vi "AlliGator Save Phasor Ratio References.vi"(8 "Error In":errorcluster) -> (0 "Error Out":errorcluster, 1 "Message":string)   [LabVIEW 2021, in "AlliGator Phasor Ratio.lvlib"]
doc: "Saves phasor reference(s) - with Dialog."
uses:
  AlliGator Phasor Ratio.lvlib
  AlliGator Phasor Ratio Reference & Lifetime v2.ctl
  Phasor/Phasor (g, s).ctl
  Phasor/Phasor.lvlib
  Files/Files.lvlib
panel:
  in  "Cancel":bool
  in  "Save":bool
  in  "Save Reference 2":bool
  in  "Save Reference 1":bool
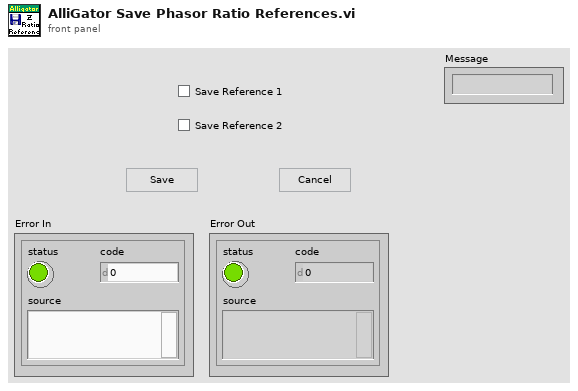
[diagram p1: front panel]
types:
  T1 = enum32{"Invalid", "Standard", "Closed", "Hidden", "Minimized", "Maximized"}
  T2 = enum8{"Enabled", "Disabled", "Disabled and Grayed Out"}
  T3 = typedef "Phasor.lvlib/Phasor (g, s).ctl" = cluster{"g":dbl, "s":dbl}
  T4 = typedef "AlliGator Phasor Ratio.lvlib/AlliGator Phasor Ratio Reference & Lifetime v2.ctl" = cluster{"Phasor Ratio Reference":T3, "Reference Lifetime":dbl[unit], "Phasor Frequency":dbl[unit]}
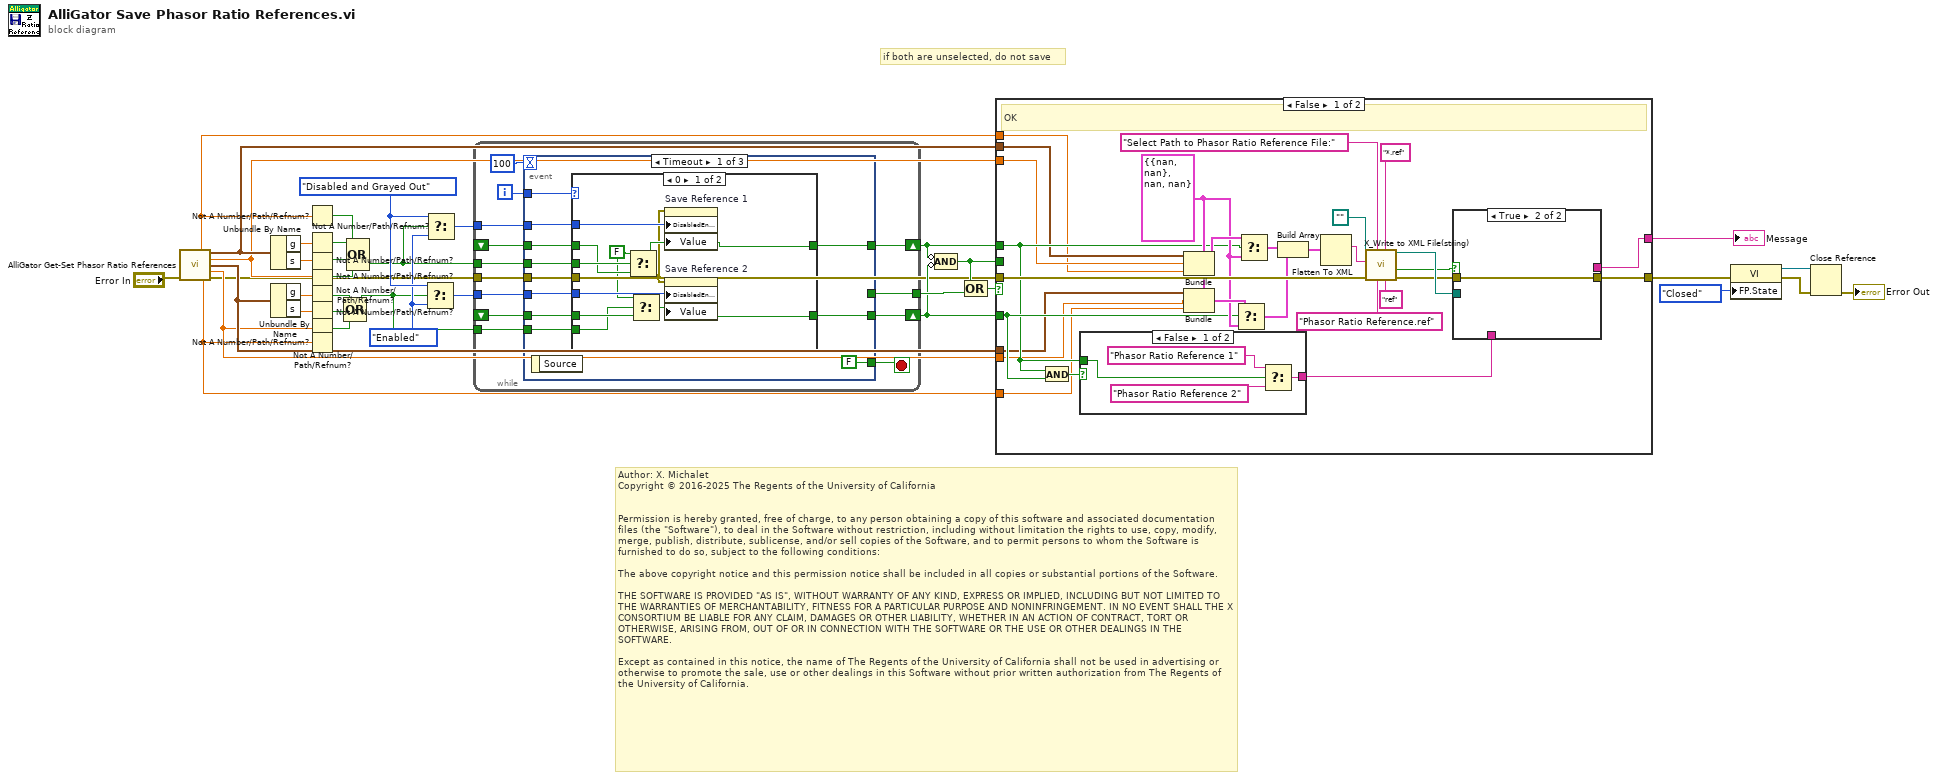
[diagram p0: block diagram]
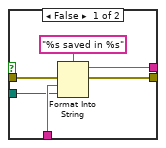
[diagram p2: hidden frame]
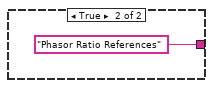
[diagram p3: hidden frame]
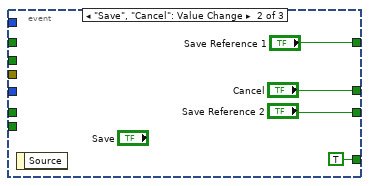
[diagram p6: hidden frame]
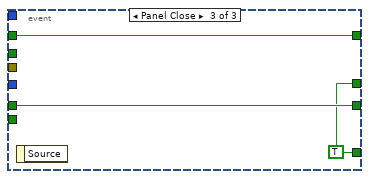
[diagram p7: hidden frame]
diagram:
  w35 = T2."Enabled" ("Disabled")
  w36 = T2."Disabled and Grayed Out" ("Disabled")
  # "Author: X. Michalet\nCopyright © 2016-2025 The Regents of the University of California\n \n\nPermission is hereby granted, free of charge, to any person obtaining a copy of this software and associated documentation files (the \"Software\"), to deal in the Software without restriction, including without limitation the rights to use, copy, modify, merge, publish, distribute, sublicense, and/or sell copies of the Software, and to permit persons to whom the Software is furnished to do so, subject to the following conditions:\n\nThe above copyright notice and this permission notice shall be included in all copies or substantial portions of the Software.\n\nTHE SOFTWARE IS PROVIDED \"AS IS\", WITHOUT WARRANTY OF ANY KIND, EXPRESS OR IMPLIED, INCLUDING BUT NOT LIMITED TO THE WARRANTIES OF MERCHANTABILITY, FITNESS FOR A PARTICULAR PURPOSE AND NONINFRINGEMENT. IN NO EVENT SHALL THE X CONSORTIUM BE LIABLE FOR ANY CLAIM, DAMAGES OR OTHER LIABILITY, WHETHER IN AN ACTION OF CONTRACT, TORT OR OTHERWISE, ARISING FROM, OUT OF OR IN CONNECTION WITH THE SOFTWARE OR THE USE OR OTHER DEALINGS IN THE SOFTWARE.\n\nExcept as contained in this notice, the name of The Regents of the University of California shall not be used in advertising or otherwise to promote the sale, use or other dealings in this Software without prior written authorization from The Regents of the University of California."
  # "if both are unselected, do not save"
  n1 = call "AlliGator Get-Set Phasor Ratio References.vi"("error in (no error)"="Error In") -> ("Reference Frequency 1"=w3:dbl[unit], "Reference Phasor 1"=w14:T3, "Reference Lifetime 1"=w13:dbl[unit], "Reference Phasor 2"=w12:T3, "Reference Lifetime 2"=w11:dbl[unit], "Reference Frequency 2"=w2:dbl[unit], "error out"=w9:errorcluster)  [unwired: 7 in, 1 out]
  n2 = Unbundle By Name(w14) -> ("g"=w18:dbl, "s"=w17:dbl)
  n3 = Unbundle By Name(w12) -> ("g"=w16:dbl, "s"=w15:dbl)
  n4 = Not A Number/Path/Refnum?(number/path/refnum=w3) -> (NaN/Path/Refnum?=w4:bool)
  n5 = Not A Number/Path/Refnum?(number/path/refnum=w18) -> (NaN/Path/Refnum?=w24:bool)
  n6 = Not A Number/Path/Refnum?(number/path/refnum=w17) -> (NaN/Path/Refnum?=w26:bool)
  n7 = Not A Number/Path/Refnum?(number/path/refnum=w13) -> (NaN/Path/Refnum?=w25:bool)
  n8 = Not A Number/Path/Refnum?(number/path/refnum=w16) -> (NaN/Path/Refnum?=w21:bool)
  n9 = Not A Number/Path/Refnum?(number/path/refnum=w15) -> (NaN/Path/Refnum?=w22:bool)
  n10 = Not A Number/Path/Refnum?(number/path/refnum=w11) -> (NaN/Path/Refnum?=w20:bool)
  n11 = Not A Number/Path/Refnum?(number/path/refnum=w2) -> ()  [unwired: 1 out]
  n12 = Compound Arithmetic op=OR(w21, w22, w20) -> (w19:bool)
  n13 = Compound Arithmetic op=OR(w4, w24, w26, w25) -> (w23:bool)
  n14 = Select(t=w36, s=w19, f=w35) -> (s? t:f=w33:T2)
  n15 = Select(t=w36, s=w23, f=w35) -> (s? t:f=w34:T2)
  n16 = while {
    tunnel: w34 -> [w49]
    tunnel: w33 -> [w48]
    shift-right: [w43] -> w29
    shift-left: _ -> [w46]
    tunnel: w23 -> [w47]
    shift-right: [w42] -> w28
    shift-left: _ -> [w40]
    tunnel: w19 -> [w41]
    tunnel: [w38] -> w32
    tunnel: w9 -> [w37]
    i -> [w44]
    stop <- w39 stop-if-true
    n17 = event shown="[0] Timeout" {
      selector: _ -> [_ _ _]
      dyn-events: _ -> [_ _ _]
      timeout: 100 -> [_ _ _]
      tunnel: w49 -> [w60 _ _]
      tunnel: w48 -> [w59 _ _]
      tunnel: w47 -> [w58 _ _]
      tunnel: w46 -> [w57 _ w79]
      tunnel: w44 -> [w56 _ _]
      tunnel: [w55 "Save Reference 1" w79] -> w43
      tunnel: [w54 "Save Reference 2" w78] -> w42
      tunnel: w41 -> [w52 _ _]
      tunnel: w40 -> [w53 _ w78]
      tunnel: [FALSE TRUE w77] -> w39
      tunnel: [_ "Cancel" w77] -> w38
      tunnel: w37 -> [w50 _ _]
      event Timeout {
        n18 = event-data() -> ()  [unwired: 1 in, 1 out]
        n19 = case shown="0" w56 {
          tunnel: w60 -> [w70 _]
          tunnel: w59 -> [w69 _]
          tunnel: w58 -> [w68 _]
          tunnel: w57 -> [w67 w72]
          tunnel: [w66 w72] -> w55
          tunnel: [w62 w71] -> w54
          tunnel: w53 -> [w64 w71]
          tunnel: w52 -> [w63 _]
          tunnel: w50 -> [w61 _]
          frame 0 {
            w65 = FALSE
            n20 = Select(t=w65, s=w68, f=w67) -> (s? t:f=w66:bool)
            n21 = Select(t=w65, s=w63, f=w64) -> (s? t:f=w62:bool)
            n22 = property on="Save Reference 1" class="Bool (strict)"(error in=w61, "DisabledEnum"=w70, "Value"=w66) -> ()  [unwired: 1 in, 2 out]
            n23 = property on="Save Reference 2" class="Bool (strict)"(error in=w61, "DisabledEnum"=w69, "Value"=w62) -> ()  [unwired: 1 in, 2 out]
          }
          frame 1, Default {
          }
        }
      }
      event "Save", "Cancel": Value Change {
        n24 = event-data() -> ()  [unwired: 1 in, 1 out]
      }
      event Panel Close {
        w77 = TRUE
        n25 = event-data() -> ()  [unwired: 1 in, 1 out]
      }
    }
  }
  n26 = Compound Arithmetic op=AND(invert w29, invert w28) -> (w27:bool)
  n27 = Compound Arithmetic op=OR(w27, w32) -> (w30:bool)
  n28 = case shown="False" w30 {
    tunnel: [w92 w120] -> w8
    tunnel: w9 -> [w107 w120]
    tunnel: w29 -> [w96 _]
    tunnel: w28 -> [w98 _]
    tunnel: w27 -> [_ _]
    tunnel: w14 -> [w88 _]
    tunnel: w13 -> [w87 _]
    tunnel: w12 -> [w86 _]
    tunnel: w11 -> [w85 _]
    tunnel: w3 -> [w84 _]
    tunnel: w2 -> [w83 _]
    tunnel: [w82 _] -> w1
    frame False {
      w99 = T4 {"Phasor Ratio Reference"={"g"=nan, "s"=nan}, "Reference Lifetime"=nan, "Phasor Frequency"=nan}
      # "OK"
      n29 = And(x=w96, y=w98) -> (x .and. y?=w97:bool)
      n30 = case shown="False" w97 {
        tunnel: w96 -> [w118 _]
        tunnel: [w115 "Phasor Ratio References" ("format string")] -> w95
        frame False {
          n31 = Select(t="Phasor Ratio Reference 1" ("format string"), s=w118, f="Phasor Ratio Reference 2" ("format string")) -> (s? t:f=w115:string)
        }
        frame True {
        }
      }
      n32 = Bundle(cluster=w99, "Phasor Ratio Reference"=w88, "Reference Lifetime"=w87, "Phasor Frequency"=w84) -> (w100:T4)
      n33 = Bundle(cluster=w99, "Phasor Ratio Reference"=w86, "Reference Lifetime"=w85, "Phasor Frequency"=w83) -> (w104:T4)
      n34 = Select(t=w104, s=w98, f=w99) -> (s? t:f=w102:T4)
      n35 = Select(t=w100, s=w96, f=w99) -> (s? t:f=w103:T4)
      n36 = Build Array(w103, w102) -> (w101:T4[])
      n37 = Flatten To XML(6:w101) -> (2:w105:string)
      n38 = call "X_Write to XML File(string).vi"("File Extension (xml)"="ref", "Pattern (*.xml;*.XML)"="*.ref", "default name"="Phasor Ratio Reference.ref", "Prompt"="Select Path to Phasor Ratio Reference File:", "error in (no error)"=w107, "XML Input"=w105, "XML File Start Path"=path "") -> ("error out"=w93:errorcluster, "cancelled"=w80:bool, "XML File Path"=w94:path)  [unwired: 1 in, 1 out]
      n39 = case shown="True" w80 {
        tunnel: w95 -> [w113 _]
        tunnel: w94 -> [w111 _]
        tunnel: w93 -> [w110 w114]
        tunnel: [w109 w114] -> w92
        tunnel: [w108 _] -> w82
        frame False {
          n40 = Format Into String(format string="%s saved in %s", error in=w110, w113, w111) -> (resulting string=w108:string, error out=w109:errorcluster)  [unwired: 1 in]
        }
        frame True {
        }
      }
    }
    frame True {
      # "Cancelled"
    }
  }
  "Message" <- w1
  n41 = property class="VI"(error in=w8, "FP.State"=T1."Closed" ("Front Panel Window:State")) -> (reference out=w31:refnum<vi>, error out=w7:errorcluster)  [unwired: 1 in]
  n42 = Close Reference(reference=w31, error in (no error)=w7) -> (error out=→"Error Out":errorcluster)
